vi "Read File sequencer.vi"(8 "error in (no error)":errorcluster caption="entrée d'erreur (pas d'erreur)", 10 "Type Product":string(combo), 11 "Part Number PCBA":string(combo)) -> (0 "error out":errorcluster caption="sortie d'erreur", 3 "Tableau":T1[](array[typedef]))   [LabVIEW 2020]
uses:
  Type DEF/Commande Gestion Execution Scenario.ctl
  Commun VI/TypeDef/Commande Test/Commande Value Type.ctl
  Commun VI/TypeDef/Commande Test/Commande Type Test.ctl
  Commun VI/Library Commun.lvlib
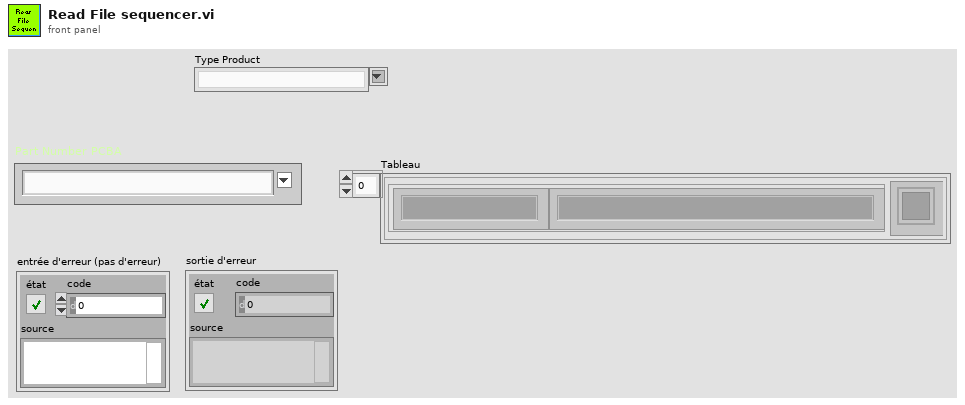
[diagram p1: front panel]
types:
  T1 = typedef "Commande Gestion Execution Scenario.ctl" = cluster{"Name Test":string, "Etat":cluster{"Menu déroulant":u16}, "Affiche result":bool, "Tab Test Result":cluster{"Main Test":string, "Name Test":string, "StartOfTest":string, "Value":string, "Limit_Low":string, "Limit_High":string, "Result":bool, "Fatal_Test":bool, "NbRetry":dbl, "EndOfTest":string, "Error":string, "TypeValue":T2, "Type Test":T3}[], "State Test":string}
  T2 = typedef "Library Commun.lvlib/Commande Value Type.ctl" = enum16{"None", "String", "Number", "Timestamp", "Boolean", "Array"}
  T3 = typedef "Library Commun.lvlib/Commande Type Test.ctl" = enum16{"Function", "Test", "Calculation"}
  T4 = cluster{"Group Name":string, "Tab Test":cluster{"Type Function":string, "Test Name":string, "Class launched by the actors ":string, "Name_Instrument":string, "Class_Instrument":string, "Parameter (Json)":string, "Limit_Low":string, "Limit_Hight":string, "Fatal Test ?":bool, "Parallelized ?":bool, "Mandatory ?":bool}[], "Parallelized ?":bool, "Mandatory ?":bool}[]
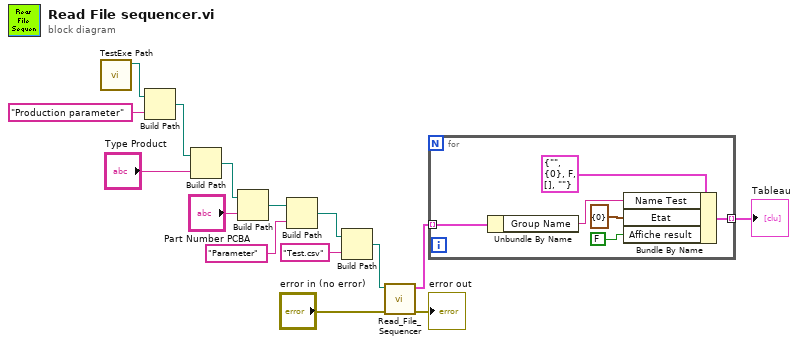
[diagram p0: block diagram]
diagram:
  n1 = call "TestExe Path.vi"() -> ("Chemin Actuel"=w8:path)  [unwired: 9 in, 2 out]
  n2 = Build Path(base path=w8, name or relative path="Production parameter" ("nom ou chemin relatif")) -> (appended path=w7:path)
  n3 = Build Path(base path=w7, name or relative path="Type Product") -> (appended path=w6:path)
  n4 = Build Path(base path=w6, name or relative path="Part Number PCBA") -> (appended path=w5:path)
  n5 = Build Path(base path=w5, name or relative path="Parameter" ("nom ou chemin relatif")) -> (appended path=w3:path)
  n6 = Build Path(base path=w3, name or relative path="Test.csv" ("nom ou chemin relatif")) -> (appended path=w15:path)
  n7 = call "Read_File_Sequencer.vi"("error in (no error)"="error in (no error)", "file path (dialog if empty)"=w15) -> ("error out"=→"error out":errorcluster, "Test Sequence"=w13:T4)  [unwired: 8 in]
  n8 = for {
    tunnel: w13 -> [w19] mode=indexing
    tunnel: [w16] -> w10 mode=indexing
    n9 = Unbundle By Name(w19) -> ("Group Name"=w20:string)
    n10 = Bundle By Name(cluster=T1 {"Name Test"="", "Etat"={"Menu déroulant"=0}, "Affiche result"=FALSE, "Tab Test Result"=[], "State Test"=""} ("ExécutionScénario_GestionScénario"), "Name Test"=w20, "Etat"=cluster{"Menu déroulant":u16} {"Menu déroulant"=0}, "Affiche result"=FALSE) -> (w16:T1)
  }
  "Tableau" <- w10
